vi "Open File Stream.vi"(0 "video in":refnum<class "MSC Video.lvclass">, 1 "File Path":path, 5 "error in (no error)":errorcluster) -> (14 "video out":refnum<class "MSC Video.lvclass">, 19 "error out":errorcluster)   [LabVIEW 2014, in "MSC Video.lvclass"]
doc: "Starts a video file stream from the selected path."
uses:
  MSC Video.lvclass
  MSC Video.lvclass/MSC Video.ctl
  Dependencies/x86/MSC I Process32.dll
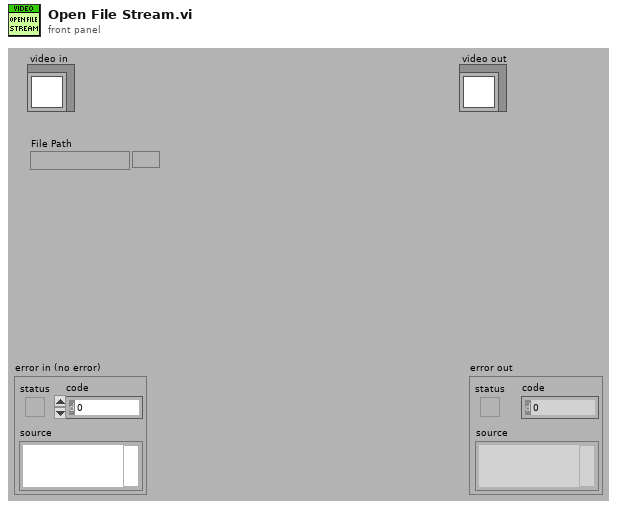
[diagram p1: front panel]
types:
  T1 = typedef "MSC Video.lvclass/Video.ctl" = cluster{"Pointer":u64, "CamID":i32, "File Path":path, "Network Address":string, "opened":bool}
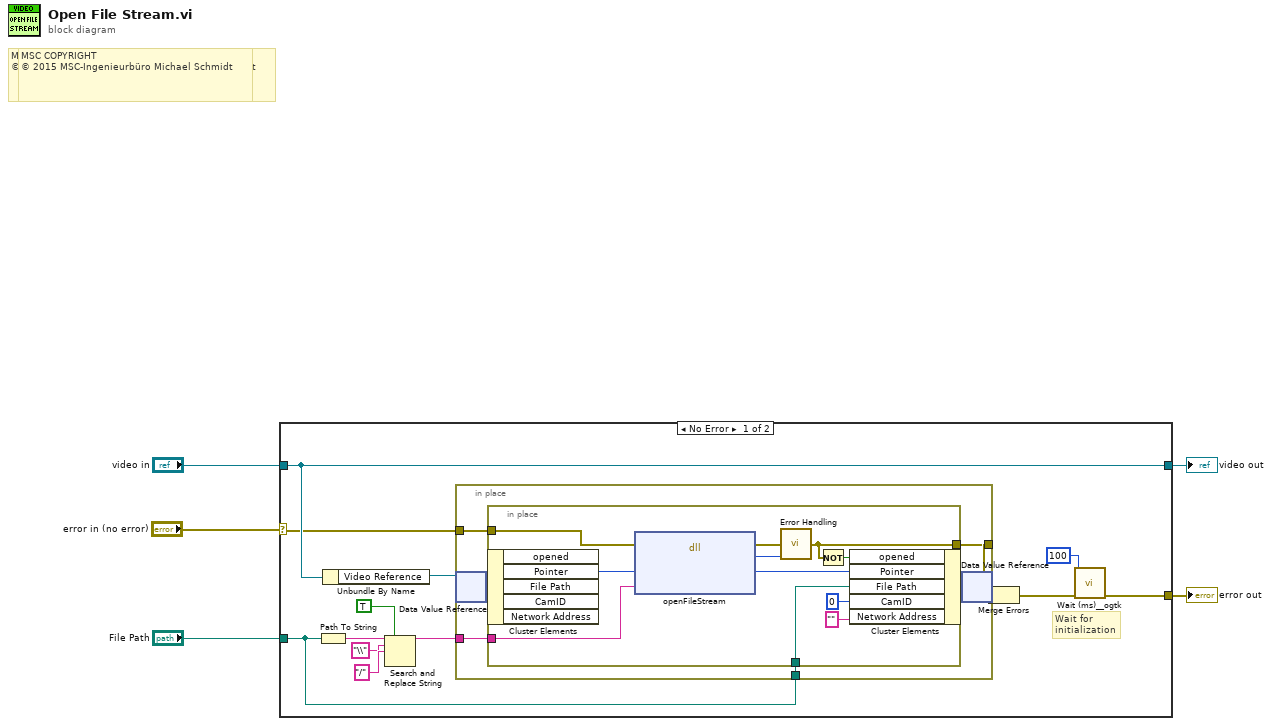
[diagram p0: block diagram]
diagram:
  # "MSC COPYRIGHT\n© 2016 MSC-Ingenieurbüro Michael Schmidt"
  # "MSC COPYRIGHT\n© 2016 MSC-Ingenieurbüro Michael Schmidt"
  # "MSC COPYRIGHT\n© 2015 MSC-Ingenieurbüro Michael Schmidt"
  n1 = case shown="No Error" "error in (no error)" {
    selector: "error in (no error)" -> [w15 w38]
    tunnel: [w14 w38] -> w4
    tunnel: "video in" -> [w16 w37]
    tunnel: [w16 w37] -> w2
    tunnel: "File Path" -> [w6 _]
    frame No Error {
      # "Wait for\ninitialization"
      n2 = Path To String(path=w6) -> (string=w11:string)
      n3 = Unbundle By Name(w16) -> ("Video Reference"=w17:refnum<data-value>)
      n4 = Search and Replace String(replace all?=TRUE ("replace all? (F)"), input string=w11, search string="\\", replace string="/" ("replace string (\"\")")) -> (result string=w7:string)  [unwired: 4 in, 3 out]
      n5 = in-place {
        in-place-border: [w23] -> w18
        in-place-border: w7 -> [w22]
        in-place-border: w15 -> [w21]
        in-place-border: w6 -> [w20]
        n6 = in-place-dvr #1(w17) -> (w24:T1)  [unwired: 1 out]
        n7 = in-place {
          in-place-border: [w32] -> w23
          in-place-border: w22 -> [w35]
          in-place-border: w21 -> [w29]
          in-place-border: w20 -> [w28]
          n8 = in-place-cluster #2(w24) -> ("Pointer"=w36:u64)  [unwired: 4 out]
          n9 = dll-call lib="C:/Users/MSC/LabVIEW Projekte/LV 2014/MSC I-Process/user.lib/MSC-I Process/Dependencies/x86/MSC I Process*.dll" fn="openFileStream"(error in=w29, "pointer"=w36, "fileString"=w35) -> (error out=w34:errorcluster, "error"=w33:i32, "pointer"=w30:u64)  [unwired: 3 in, 1 out]
          n10 = call "Error Handling.vi"("error in (no error)"=w34, "return type"=w33) -> ("error out"=w32:errorcluster)  [unwired: 12 in, 1 out]
          n11 = Not(x=w32) -> (.not. x?=w31:bool)
          n12 = in-place-cluster #2("opened"=w31, "Pointer"=w30, "File Path"=w28, "CamID"=0, "Network Address"="") -> (w25:T1)
        }
        n13 = in-place-dvr #1(w25) -> (w19:errorcluster)  [unwired: 1 out]
      }
      n14 = Merge Errors(w18, w19) -> (w13:errorcluster)
      n15 = call <userlib>:"Wait (ms)__ogtk.vi"("error in (no error)"=w13, "milliseconds to wait"=u32 100) -> ("error out"=w14:errorcluster)  [unwired: 8 in, 1 out]
    }
    frame Error {
    }
  }
  "error out" <- w4
  "video out" <- w2
